vi "Get Temperature.vi"(11 "temperature":i32) -> (2 "function return":u32, 3 "temperature out":i32)   [LabVIEW 2018, in "AndorSDK.lvlib"]
doc: "EXPNETTYPE unsigned int WINAPI GetTemperature(int * temperature);"
uses:
  AndorSDK.lvlib
  ATMCD32D.dll
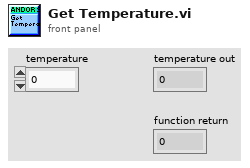
[diagram p1: front panel]
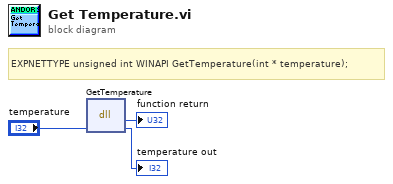
[diagram p0: block diagram]
diagram:
  # "EXPNETTYPE unsigned int WINAPI GetTemperature(int * temperature);"
  n1 = dll-call lib="PTH2babs E\nPersönliches02 - Arbeit03-HiwijobsLabviewCodelibANDOR\tAndor SDK\nATMCD32D.*" fn="GetTemperature"("temperature"="temperature") -> (→"function return":u32, "temperature"=→"temperature out":i32)  [unwired: 3 in, 2 out]
